vi "Get Instrument.vi"(8 "error in (no error)":errorcluster, 10 "Instrument Number":u32, 11 "Application in":refnum<class "Application.lvclass">) -> (0 "error out":errorcluster, 2 "Instrument":refnum<class "Instrument.lvclass">, 3 "Application out":refnum<class "Application.lvclass">)   [LabVIEW 2017, in "Application.lvlib" / "Application.lvclass"]
doc: "Retrieves an instrument from an application by number. Use the appropriate typedef to select."
uses:
  Application.lvclass
  Instruments/Instrument/Class/Instrument.lvclass
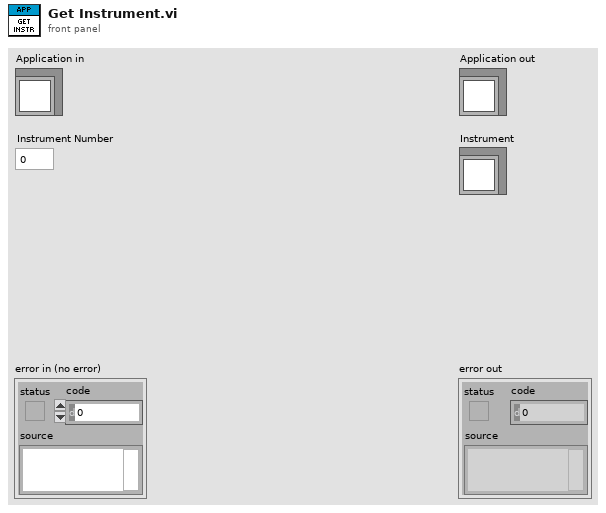
[diagram p1: front panel]
types:
  T1 = typedef "Application.lvlib/App Properties.lvclass/Class Properties -- Cluster.ctl" = cluster{"UUT Info":T2[], "Test Information":refnum<vi>, "Gold Board":refnum<class "Golden Board.lvclass">, "Test Recipe":refnum<class "Test Recipe.lvclass">, "Instruments":refnum<class "Instrument.lvclass">[], "Mode":T3, "Test Results":T4[], "Station Config":refnum<class "Station Config.lvclass">, "Variable Engine":refnum<class "Variable Engine.lvclass">}
  T2 = typedef "Application.lvlib/App Properties.lvclass/UUT Reference -- Cluster.ctl" = cluster{"Serial Number Reference":refnum<vi>, "Status Message Reference":refnum<vi>}
  T3 = typedef "Application.lvlib/Application.lvclass/Op Mode -- Enum.ctl" = u16
  T4 = typedef "Application.lvlib/App Properties.lvclass/Test Result -- Cluster.ctl" = cluster{"Position":i32, "Pass":bool, "Fail Codes":string}
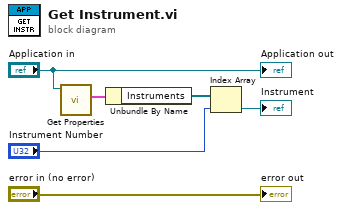
[diagram p0: block diagram]
diagram:
  n1 = call "Get Properties.vi"("Acrobat Template in"="Application in") -> ("Class Properties"=w4:T1)  [unwired: 8 in, 2 out]
  n2 = Unbundle By Name(w4) -> ("Instruments"=w3:refnum<class "Instrument.lvclass">[])
  n3 = Index Array(array=w3, index="Instrument Number") -> (element=→"Instrument":refnum<class "Instrument.lvclass">)
  "error out" <- "error in (no error)"
  "Application out" <- "Application in"
